vi "XY Sub_VI.vi"(3 "error in (no error)":errorcluster, 5 "XY Cluster In":T1 {"Y Data"."Input"."Tol" min=0.0; "X Data"."Input"."Tol" min=0.0}) -> (0 "error out":errorcluster, 2 "XY Cluster Out":T1 {"Y Data"."Input"."Tol" min=0.0; "X Data"."Input"."Tol" min=0.0})   [LabVIEW 2017]
uses:
  Encoder Cluster.ctl
  <vilib>/myRIO/Common/Instrument Driver Framework/myRIO v1.0/Encoder/typedefs/Encoder Count Direction Enum.ctl
  XY Cluster.ctl
  Motor Status Enum.ctl
  Motion Type Def.ctl
  <vilib>/addons/control/pid/pid.llb/PID Control Input Filter (DBL).vi
  <vilib>/addons/control/pid/pid.llb/PID (DBL).vi
  <vilib>/addons/control/pid/NI_PID_pid.lvlib
  <vilib>/ptbypt/NI_PtbyPt.lvlib
panel:
  out "Data Array":string[][](array[string])
  out "Stop":bool
  out "Y dist > +20":bool
  out "X dist > +20":bool
  out "X V Array":dbl[](array[numeric])
  out "Y V Array":dbl[](array[numeric])
  out "Encoder Output":T4
  out "X&Y Complete":bool
  out "Y PID Output":dbl format="%.2f"
  out "X PID Output":dbl format="%.2f"
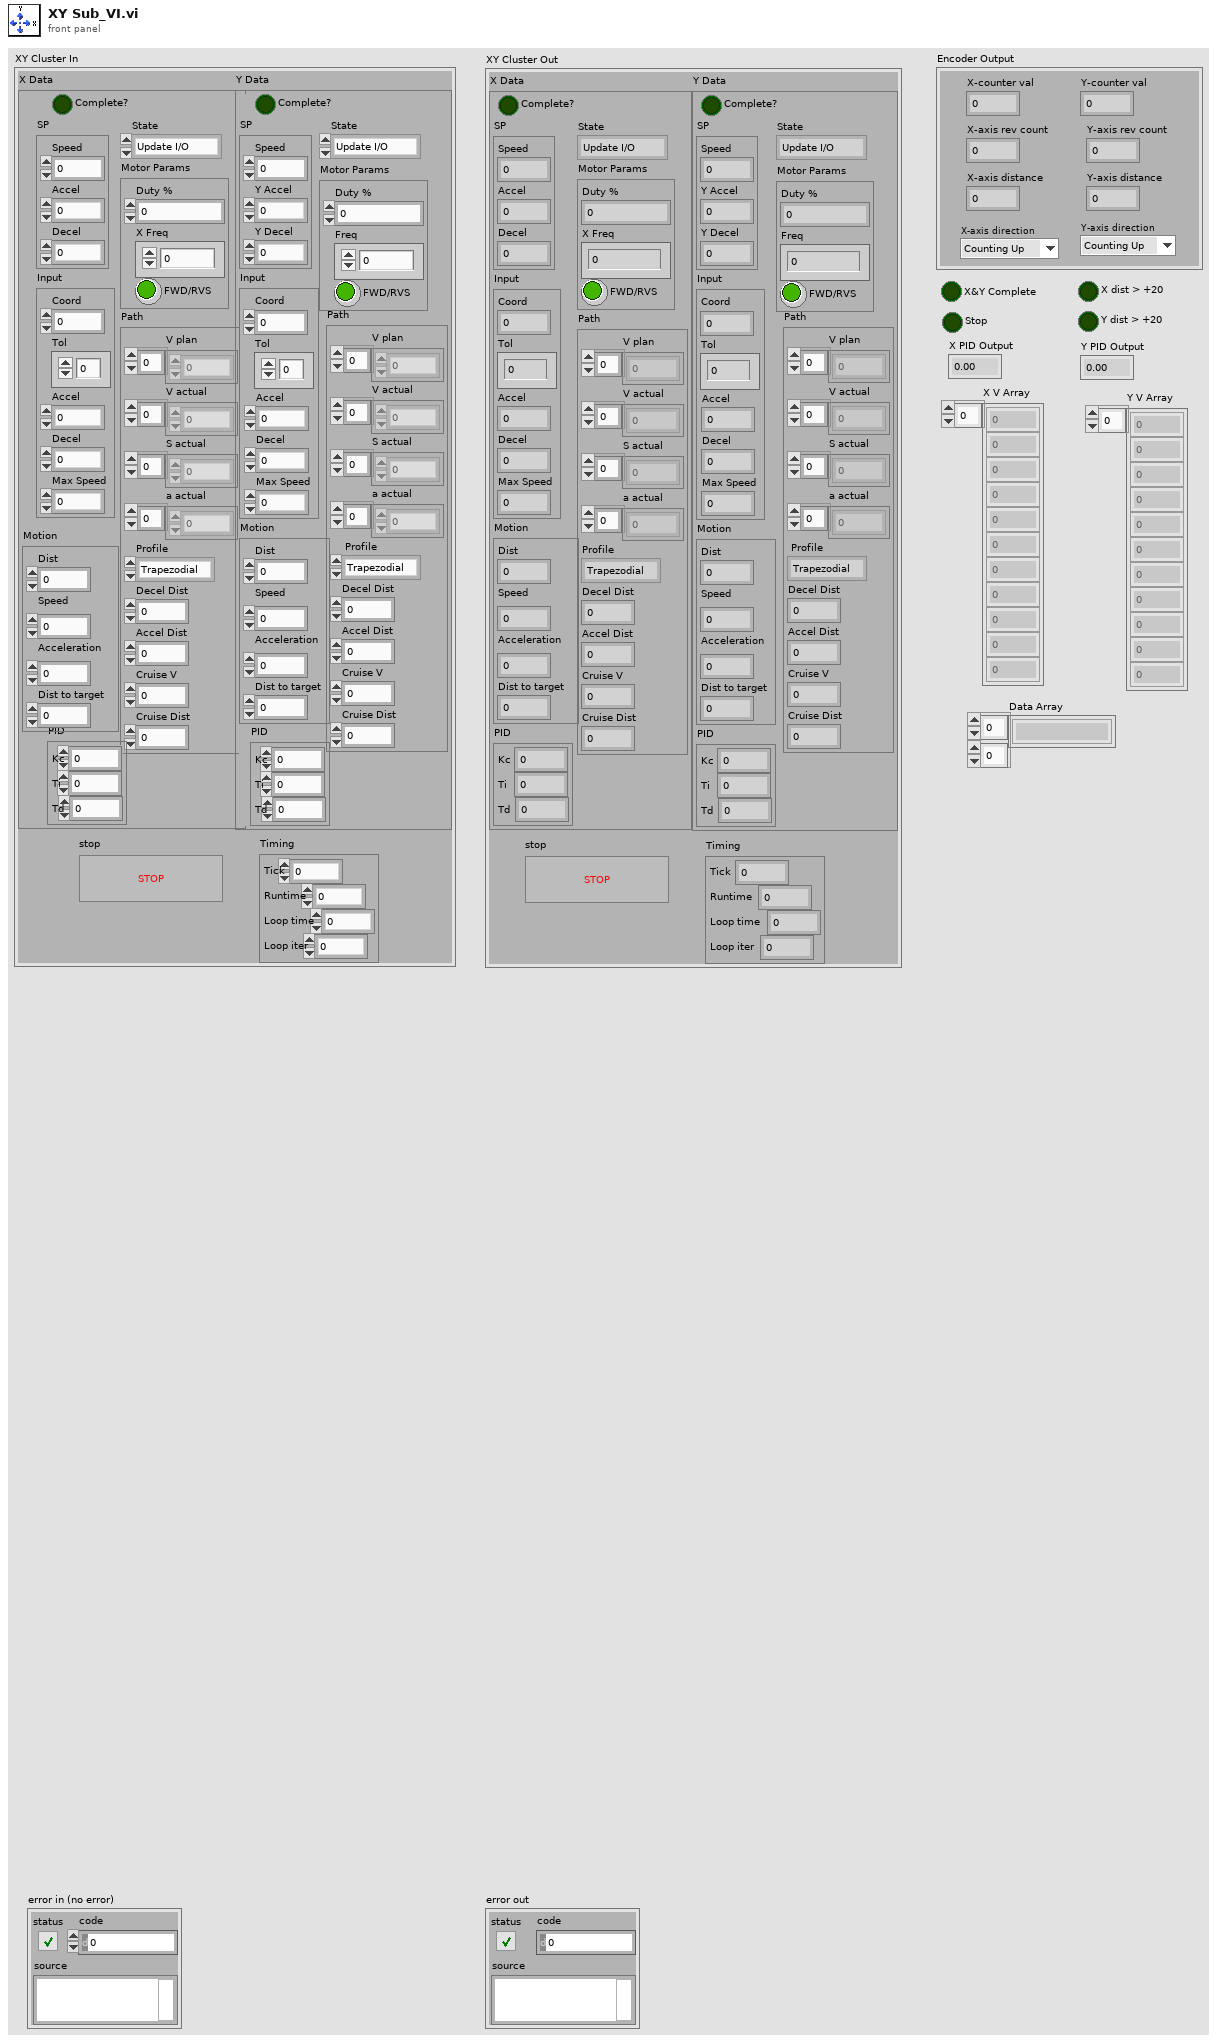
[diagram p1: front panel]
types:
  T1 = typedef "XY Cluster.ctl" = cluster{"X Data":cluster{"Complete?":bool, "Motor Params":cluster{"Duty %":dbl, "X Freq":dbl, "FWD/RVS":bool}, "SP":cluster{"Accel":dbl, "Decel":dbl, "Speed":dbl}, "State":T2, "Input":cluster{"Coord":dbl, "Tol":dbl, "Accel":dbl, "Decel":dbl, "Max Speed":dbl}, "Path":cluster{"V plan":dbl[], "V actual":dbl[], "S actual":dbl[], "a actual":dbl[], "Profile":T3, "Decel Dist":dbl, "Accel Dist":dbl, "Cruise V":dbl, "Cruise Dist":dbl}, "PID":cluster{"Kc":dbl, "Ti":dbl, "Td":dbl}, "Motion":cluster{"Speed":dbl, "Dist":dbl, "Acceleration":dbl, "Dist to target":dbl}}, "Y Data":cluster{"Complete?":bool, "Motor Params":cluster{"Duty %":dbl, "Freq":dbl, "FWD/RVS":bool}, "SP":cluster{"Y Accel":dbl, "Y Decel":dbl, "Speed":dbl}, "State":T2, "Input":cluster{"Coord":dbl, "Tol":dbl, "Accel":dbl, "Decel":dbl, "Max Speed":dbl}, "Path":cluster{"V plan":dbl[], "V actual":dbl[], "S actual":dbl[], "a actual":dbl[], " Profile":T3, "Decel Dist":dbl, "Accel Dist":dbl, "Cruise V":dbl, "Cruise Dist":dbl}, "PID":cluster{"Kc":dbl, "Ti":dbl, "Td":dbl}, "Motion":cluster{"Speed":dbl, "Dist":dbl, "Acceleration":dbl, "Dist to target":dbl}}, "Timing":cluster{"Runtime":dbl, "Loop time":dbl, "Loop iter":i32, "Tick":dbl}, "stop":bool}
  T2 = typedef "Motor Status Enum.ctl" = enum16{"Update I/O", "Stop", "Steady Speed", "Accelerate", "Decelerate", "Drive Motor"}
  T3 = typedef "Motion Type Def.ctl" = enum16{"Trapezodial", "Triangular"}
  T4 = typedef "Encoder Cluster.ctl" = cluster{"Y-axis rev count":dbl, "Y-axis distance":dbl, "X-axis rev count":dbl, "X-axis distance":dbl, "Y-axis direction":T5, "X-axis direction":T5, "X-counter val":i32, "Y-counter val":i32}
  T5 = typedef "Encoder Count Direction Enum.ctl" = enum16{"Counting Up", "Counting Down"}
  T6 = cluster{"Dist to target (mm)":dbl, "Max Speed (mm/s)":dbl, "Max Accel (mm/s^2)":dbl, "Max Decel (mm/s^2)":dbl, "Step Time (s)":dbl}
  T7 = cluster{" Distance target (mm)":dbl, "Max Accel (mm/s^2)":dbl, "Max Decel (mm/s^2)":dbl, "Velocity Limit (mm/s) ":dbl}
  T8 = cluster{"Complete?":bool, "Motor Params":cluster{"Duty %":dbl, "X Freq":dbl, "FWD/RVS":bool}, "SP":cluster{"Accel":dbl, "Decel":dbl, "Speed":dbl}, "State":T2, "Input":cluster{"Coord":dbl, "Tol":dbl, "Accel":dbl, "Decel":dbl, "Max Speed":dbl}, "Path":cluster{"V plan":dbl[], "V actual":dbl[], "S actual":dbl[], "a actual":dbl[], "Profile":T3, "Decel Dist":dbl, "Accel Dist":dbl, "Cruise V":dbl, "Cruise Dist":dbl}, "PID":cluster{"Kc":dbl, "Ti":dbl, "Td":dbl}, "Motion":cluster{"Speed":dbl, "Dist":dbl, "Acceleration":dbl, "Dist to target":dbl}}
  T9 = cluster{"Crusing Time (s)":dbl, "Decel Time (s)":dbl, "Accel Time (s)":dbl, "Total Time (s)":dbl, "Accel Distance (mm)":dbl, "Decel Distance (mm)":dbl, "Crusing Distance (mm)":dbl, "Total Dist (mm)":dbl, "Max Speed (mm/s)":dbl}
  T10 = cluster{"Complete?":bool, "Motor Params":cluster{"Duty %":dbl, "Freq":dbl, "FWD/RVS":bool}, "SP":cluster{"Y Accel":dbl, "Y Decel":dbl, "Speed":dbl}, "State":T2, "Input":cluster{"Coord":dbl, "Tol":dbl, "Accel":dbl, "Decel":dbl, "Max Speed":dbl}, "Path":cluster{"V plan":dbl[], "V actual":dbl[], "S actual":dbl[], "a actual":dbl[], " Profile":T3, "Decel Dist":dbl, "Accel Dist":dbl, "Cruise V":dbl, "Cruise Dist":dbl}, "PID":cluster{"Kc":dbl, "Ti":dbl, "Td":dbl}, "Motion":cluster{"Speed":dbl, "Dist":dbl, "Acceleration":dbl, "Dist to target":dbl}}
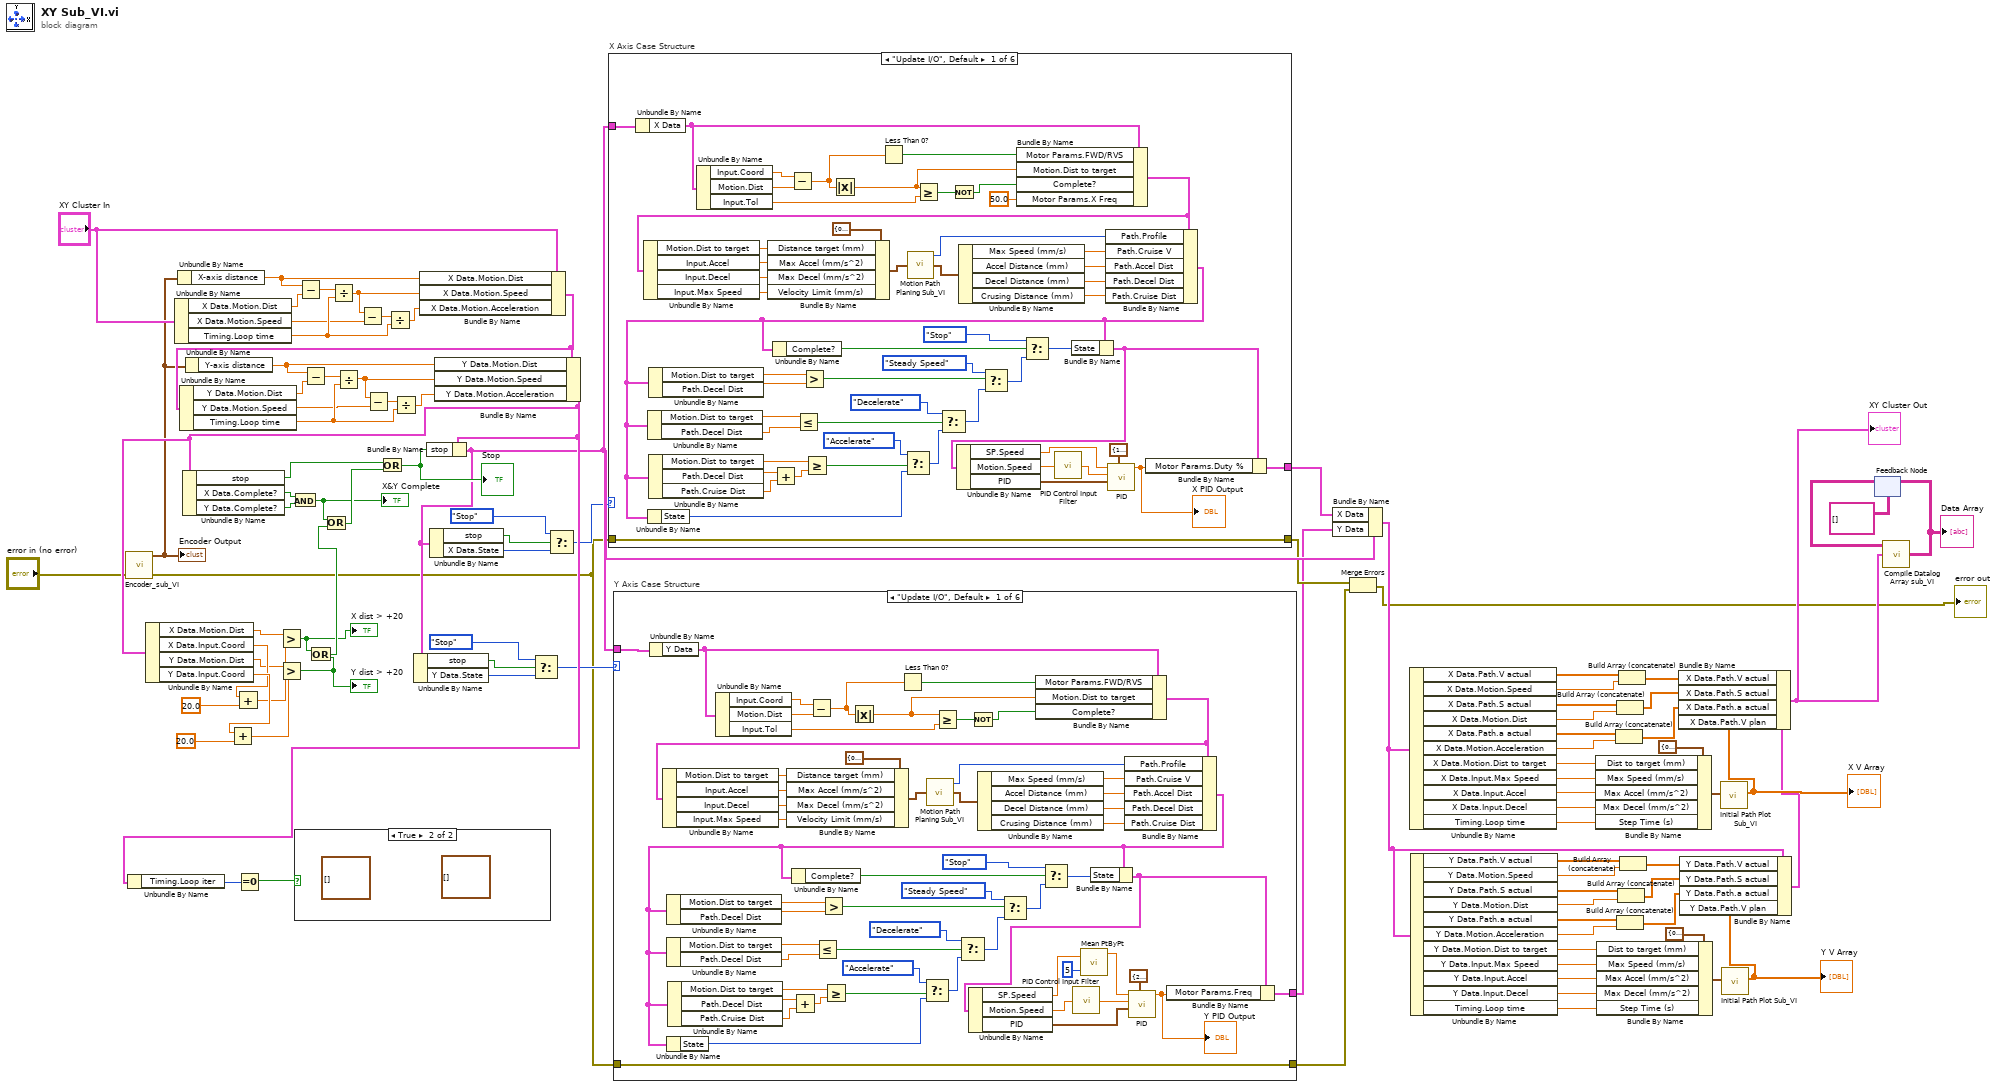
[diagram p0: block diagram]
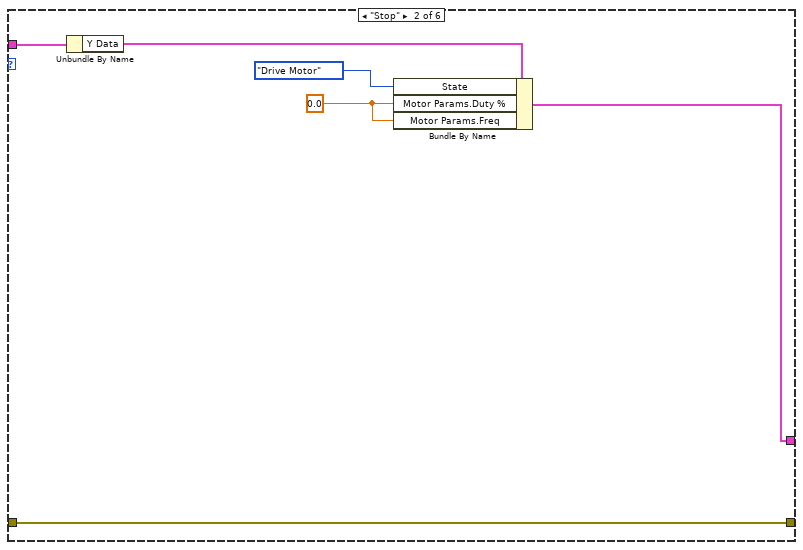
[diagram p3: hidden frame]
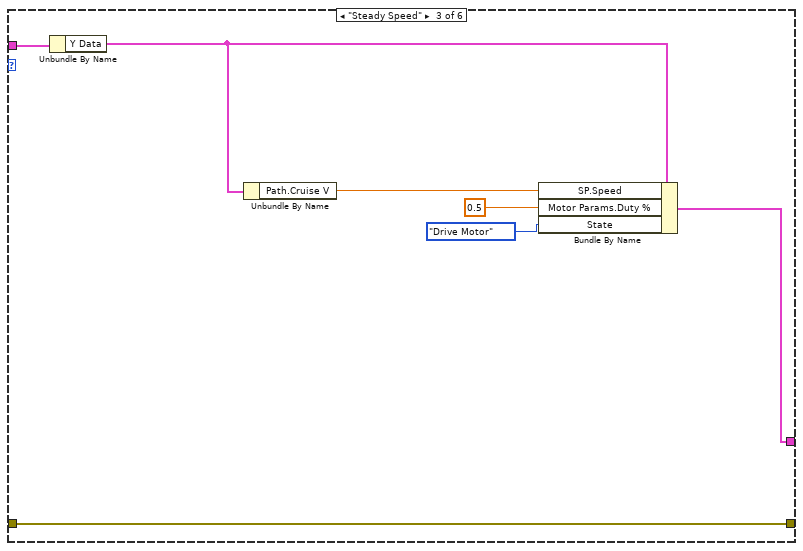
[diagram p4: hidden frame]
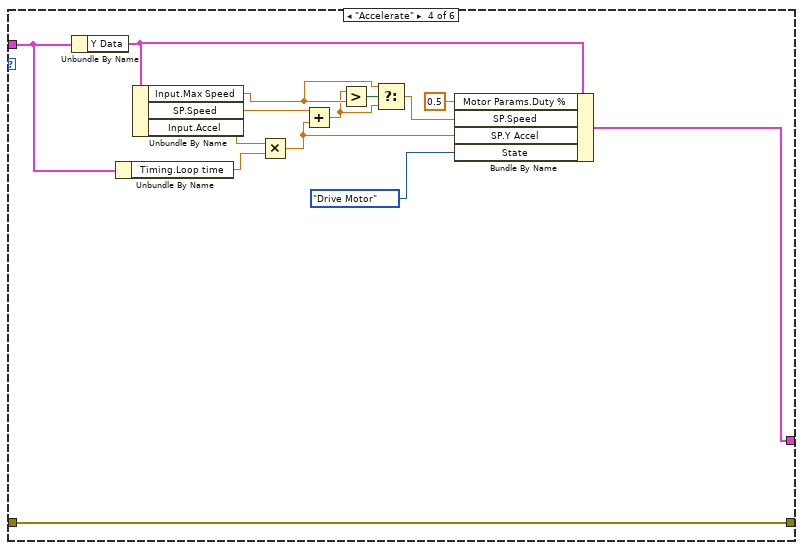
[diagram p5: hidden frame]
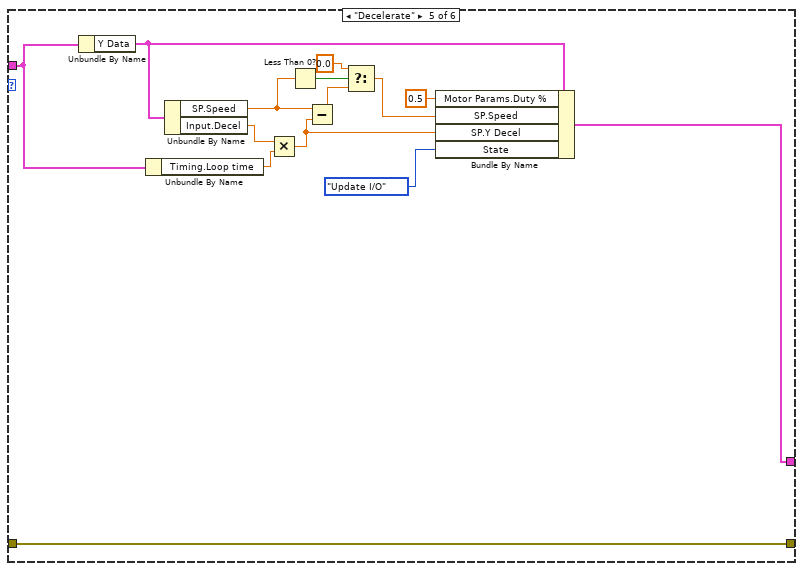
[diagram p6: hidden frame]
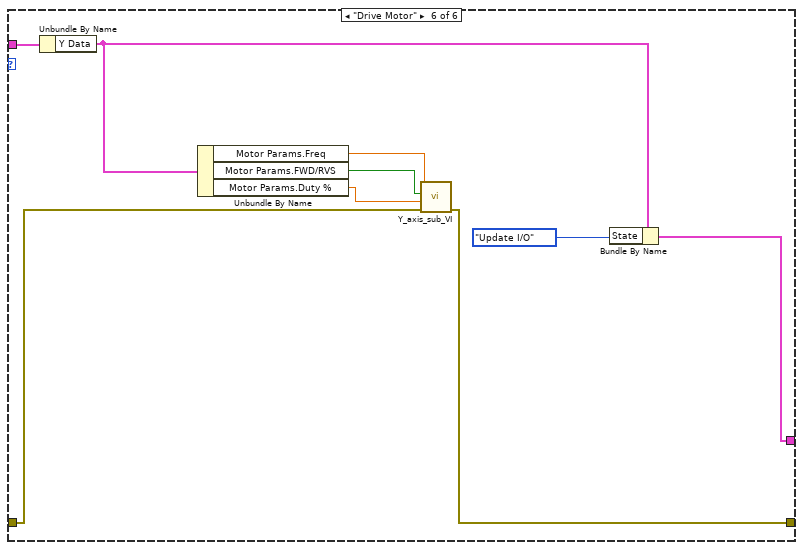
[diagram p7: hidden frame]
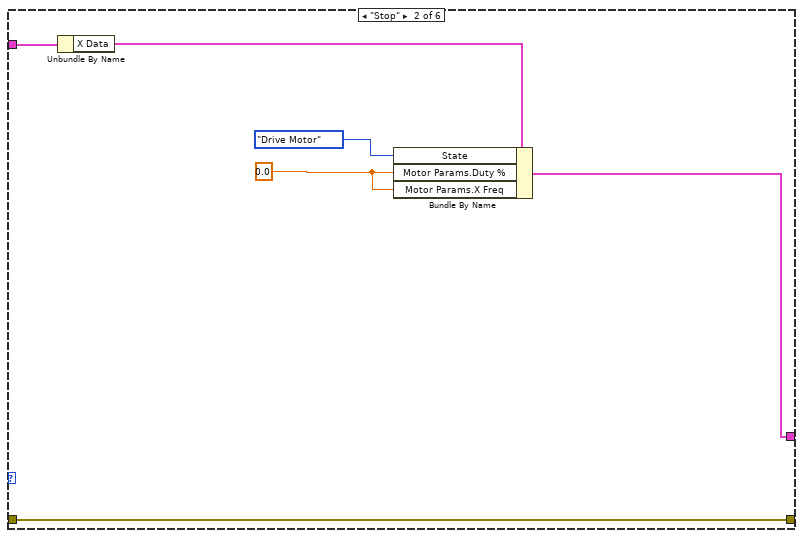
[diagram p8: hidden frame]
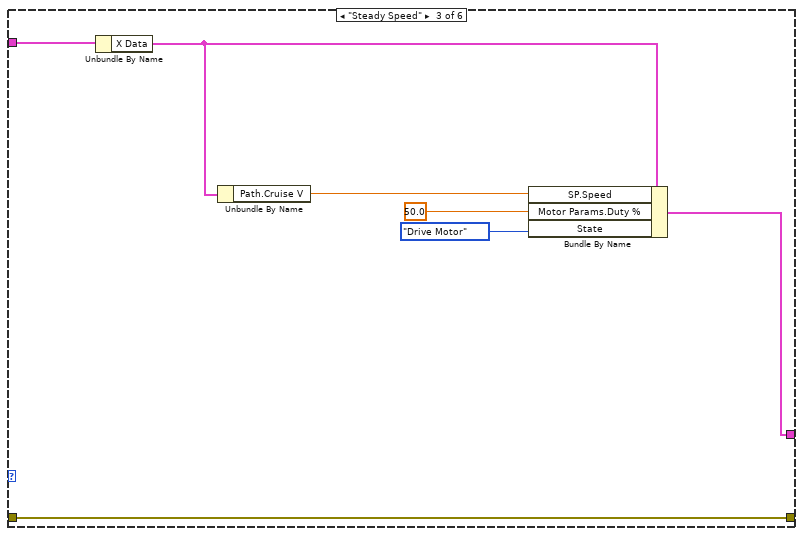
[diagram p9: hidden frame]
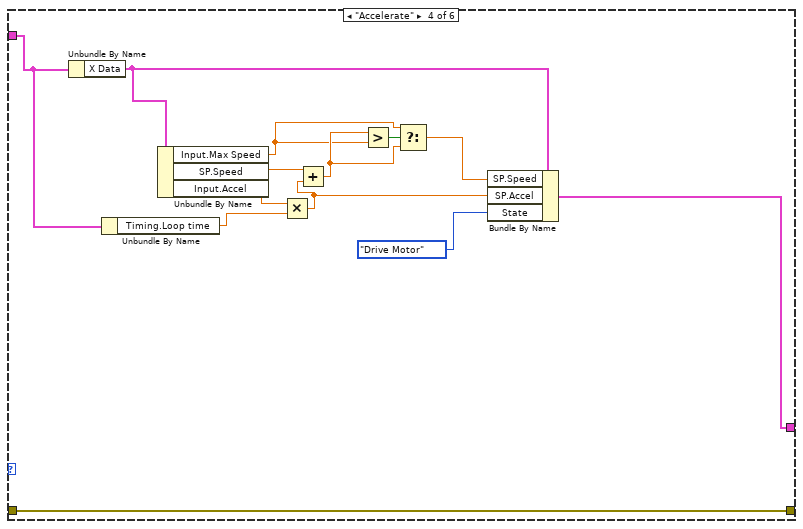
[diagram p10: hidden frame]
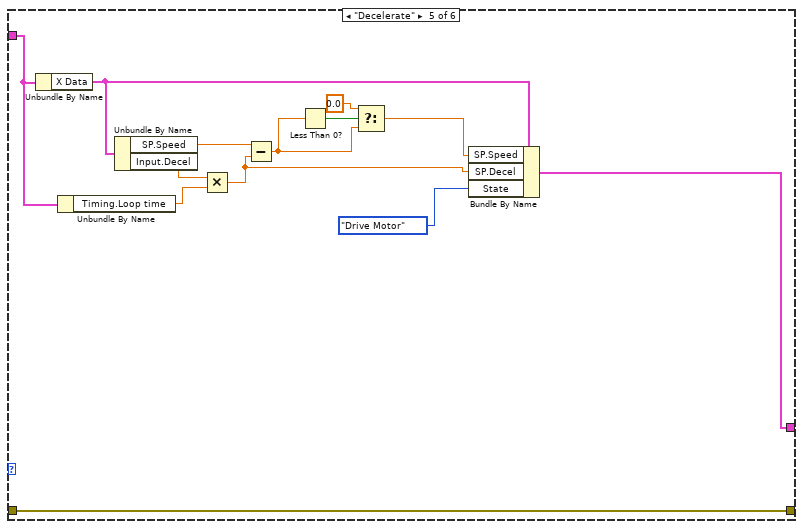
[diagram p11: hidden frame]
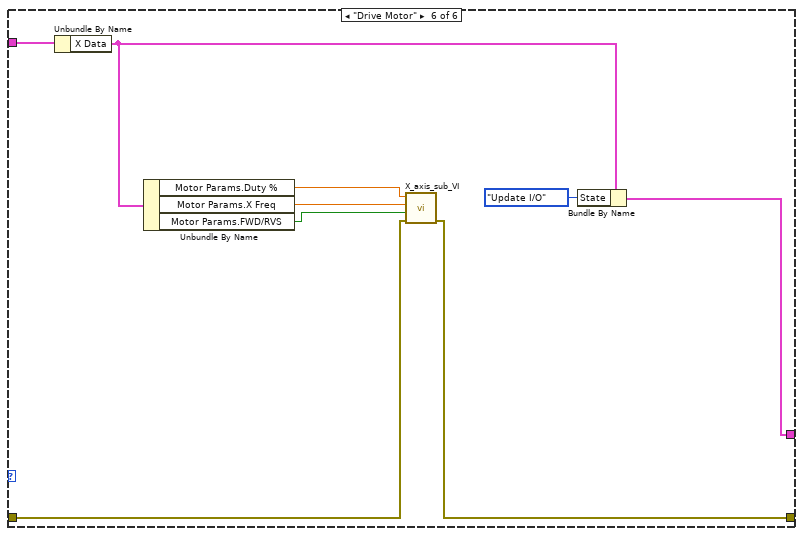
[diagram p12: hidden frame]
diagram:
  n1 = call "Encoder_sub_VI.vi"("error in (no error)"="error in (no error)") -> ("error out"=w22:errorcluster, "Encoder Output"=w12:T4)  [unwired: 9 in]
  "Encoder Output" <- w12
  n2 = Unbundle By Name("XY Cluster In") -> ("X Data.Motion.Dist"=w5:dbl, "X Data.Motion.Speed"=w8:dbl, "Timing.Loop time"=w10:dbl)
  n3 = Unbundle By Name(w12) -> ("X-axis distance"=w4:dbl)
  n4 = Unbundle By Name(w12) -> ("Y-axis distance"=w21:dbl)
  n5 = Subtract(x=w4, y=w5) -> (x-y=w6:dbl)
  n6 = Divide(x=w6, y=w10) -> (x/y=w9:dbl)
  n7 = Subtract(x=w9, y=w8) -> (x-y=w7:dbl)
  n8 = Divide(x=w7, y=w10) -> (x/y=w11:dbl)
  n9 = Bundle By Name(cluster="XY Cluster In", "X Data.Motion.Dist"=w4, "X Data.Motion.Speed"=w9, "X Data.Motion.Acceleration"=w11) -> (w20:T1)
  n10 = Unbundle By Name(w20) -> ("Y Data.Motion.Dist"=w13:dbl, "Y Data.Motion.Speed"=w16:dbl, "Timing.Loop time"=w18:dbl)
  n11 = Subtract(x=w21, y=w13) -> (x-y=w14:dbl)
  n12 = Divide(x=w14, y=w18) -> (x/y=w17:dbl)
  n13 = Subtract(x=w17, y=w16) -> (x-y=w15:dbl)
  n14 = Divide(x=w15, y=w18) -> (x/y=w19:dbl)
  n15 = Bundle By Name(cluster=w20, "Y Data.Motion.Dist"=w21, "Y Data.Motion.Speed"=w17, "Y Data.Motion.Acceleration"=w19) -> (w91:T1)
  n16 = Unbundle By Name(w91) -> ("Timing.Loop iter"=w93:i32)
  n17 = Unbundle By Name(w91) -> ("X Data.Motion.Dist"=w79:dbl, "X Data.Input.Coord"=w86:dbl, "Y Data.Motion.Dist"=w81:dbl, "Y Data.Input.Coord"=w89:dbl)
  n18 = Unbundle By Name(w91) -> ("stop"=w1:bool, "X Data.Complete?"=w38:bool, "Y Data.Complete?"=w39:bool)
  n19 = Add(x=w89, y=20.0) -> (x+y=w90:dbl)
  n20 = Add(x=w86, y=20.0) -> (x+y=w87:dbl)
  n21 = Equal To 0?(x=w93) -> (x = 0?=w92:bool)
  n22 = Greater?(x=w79, y=w87) -> (0:w80:bool)
  "X dist > +20" <- w80
  n23 = Greater?(x=w81, y=w90) -> (0:w84:bool)
  "Y dist > +20" <- w84
  n24 = And(x=w38, y=w39) -> (x .and. y?=w83:bool)
  "X&Y Complete" <- w83
  n25 = case shown="True" w92 {
    frame False {
    }
    frame True {
      (unwired) cluster{"Speed":dbl, "Speed":dbl}[] [] ("History Data")
      (unwired) cluster{"Speed":dbl, "Speed":dbl}[] [] ("History Data")
    }
  }
  n26 = Or(x=w80, y=w84) -> (x .or. y?=w82:bool)
  n27 = Or(x=w83, y=w82) -> (x .or. y?=w94:bool)
  n28 = Or(x=w1, y=w94) -> (x .or. y?=w95:bool)
  "Stop" <- w95
  n29 = Bundle By Name(cluster=w91, "stop"=w95) -> (w77:T1)
  n30 = Unbundle By Name(w77) -> ("stop"=w35:bool, "Y Data.State"=w34:T2)
  n31 = Unbundle By Name(w77) -> ("stop"=w31:bool, "X Data.State"=w30:T2)
  n32 = Select(t=Motor_Status_Enum."Stop", s=w35, f=w34) -> (s? t:f=w37:T2)
  n33 = Select(t=Motor_Status_Enum."Stop", s=w31, f=w30) -> (s? t:f=w33:T2)
  n34 = case "X Axis Case Structure" shown="\"Update I/O\", Default" w33 {
    tunnel: [w119 w156 w161 w175 w183 w191] -> w3
    tunnel: w22 -> [w140 w151 w159 w173 w182 w194]
    tunnel: [w140 w151 w159 w173 w182 w193] -> w25
    tunnel: w77 -> [w120 w153 w162 w174 w185 w198]
    frame "Update I/O", Default {
      n35 = Unbundle By Name(w120) -> ("X Data"=w102:T8)
      n36 = Unbundle By Name(w102) -> ("Input.Coord"=w150:dbl, "Motion.Dist"=w145:dbl, "Input.Tol"=w149:dbl)
      n37 = Subtract(x=w150, y=w145) -> (x-y=w146:dbl)
      n38 = Absolute Value(x=w146) -> (abs(x)=w117:dbl)
      n39 = Less Than 0?(x=w146) -> (x < 0?=w118:bool)
      n40 = Greater Or Equal?(x=w117, y=w149) -> (x >= y?=w148:bool)
      n41 = Not(x=w148) -> (.not. x?=w147:bool)
      n42 = Bundle By Name(cluster=w102, "Motor Params.FWD/RVS"=w118, "Motion.Dist to target"=w117, "Complete?"=w147, "Motor Params.X Freq"=50.0) -> (w115:T8)
      n43 = Unbundle By Name(w115) -> ("Motion.Dist to target"=w116:dbl, "Input.Accel"=w137:dbl, "Input.Decel"=w136:dbl, "Input.Max Speed"=w138:dbl)
      n44 = Bundle By Name(cluster=T7 {" Distance target (mm)"=0.0, "Max Accel (mm/s^2)"=0.0, "Max Decel (mm/s^2)"=0.0, "Velocity Limit (mm/s) "=0.0} ("Motion Planning Inputs"), "Distance target (mm)"=w116, "Max Accel (mm/s^2)"=w137, "Max Decel (mm/s^2)"=w136, "Velocity Limit (mm/s)"=w138) -> (w98:T7)
      n45 = call "Motion Path Planing Sub_VI.vi"("Motion Planning Inputs"=w98) -> ("Motion Profile"=w97:T3, "Motion Planning Outputs"=w96:T9)  [unwired: 5 in]
      n46 = Unbundle By Name(w96) -> ("Max Speed (mm/s)"=w139:dbl, "Accel Distance (mm)"=w134:dbl, "Decel Distance (mm)"=w133:dbl, "Crusing Distance (mm)"=w114:dbl)
      n47 = Bundle By Name(cluster=w115, "Path.Profile"=w97, "Path.Cruise V"=w139, "Path.Accel Dist"=w134, "Path.Decel Dist"=w133, "Path.Cruise Dist"=w114) -> (w109:T8)
      n48 = Unbundle By Name(w109) -> ("Motion.Dist to target"=w111:dbl, "Path.Decel Dist"=w110:dbl)
      n49 = Unbundle By Name(w109) -> ("State"=w131:T2)
      n50 = Unbundle By Name(w109) -> ("Motion.Dist to target"=w113:dbl, "Path.Decel Dist"=w112:dbl)
      n51 = Unbundle By Name(w109) -> ("Motion.Dist to target"=w105:dbl, "Path.Decel Dist"=w108:dbl, "Path.Cruise Dist"=w107:dbl)
      n52 = Unbundle By Name(w109) -> ("Complete?"=w123:bool)
      n53 = Add(x=w108, y=w107) -> (x+y=w106:dbl)
      n54 = Less Or Equal?(x=w111, y=w110) -> (x <= y?=w130:bool)
      n55 = Greater?(x=w113, y=w112) -> (0:w126:bool)
      n56 = Greater Or Equal?(x=w105, y=w106) -> (x >= y?=w104:bool)
      n57 = Select(t=Motor_Status_Enum."Accelerate" ("State"), s=w104, f=w131) -> (s? t:f=w129:T2)
      n58 = Select(t=Motor_Status_Enum."Decelerate" ("State"), s=w130, f=w129) -> (s? t:f=w125:T2)
      n59 = Select(t=Motor_Status_Enum."Steady Speed" ("State"), s=w126, f=w125) -> (s? t:f=w124:T2)
      n60 = Select(t=Motor_Status_Enum."Stop" ("State"), s=w123, f=w124) -> (s? t:f=w121:T2)
      n61 = Bundle By Name(cluster=w109, "State"=w121) -> (w103:T8)
      n62 = Unbundle By Name(w103) -> ("SP.Speed"=w135:dbl, "Motion.Speed"=w143:dbl, "PID"=w142:cluster{"Kc":dbl, "Ti":dbl, "Td":dbl})
      n63 = call-poly <vilib>:"PID Control Input Filter.vi"("input"=w143) -> ("output"=w144:dbl)  [unwired: 4 in]
      n64 = call-poly <vilib>:"PID.vi"("output range"=cluster{"output high":dbl, "output low":dbl} {"output high"=100.0, "output low"=0.0}, "PID gains"=w142, "process variable"=w144, "setpoint"=w135) -> ("output"=w101:dbl)  [unwired: 6 in, 1 out]
      "X PID Output" <- w101
      n65 = Bundle By Name(cluster=w103, "Motor Params.Duty %"=w101) -> (w119:T8)
    }
    frame "Stop" {
      w155 = 0.0
      n66 = Unbundle By Name(w153) -> ("X Data"=w152:T8)
      n67 = Bundle By Name(cluster=w152, "State"=Motor_Status_Enum."Drive Motor", "Motor Params.Duty %"=w155, "Motor Params.X Freq"=w155) -> (w156:T8)
    }
    frame "Steady Speed" {
      n68 = Unbundle By Name(w162) -> ("X Data"=w158:T8)
      n69 = Unbundle By Name(w158) -> ("Path.Cruise V"=w157:dbl)
      n70 = Bundle By Name(cluster=w158, "SP.Speed"=w157, "Motor Params.Duty %"=50.0, "State"=Motor_Status_Enum."Drive Motor") -> (w161:T8)
    }
    frame "Accelerate" {
      n71 = Unbundle By Name(w174) -> ("X Data"=w176:T8)
      n72 = Unbundle By Name(w174) -> ("Timing.Loop time"=w172:dbl)
      n73 = Unbundle By Name(w176) -> ("Input.Max Speed"=w164:dbl, "SP.Speed"=w170:dbl, "Input.Accel"=w169:dbl)
      n74 = Multiply(x=w169, y=w172) -> (x*y=w168:dbl)
      n75 = Add(x=w170, y=w168) -> (x+y=w165:dbl)
      n76 = Greater?(x=w165, y=w164) -> (0:w167:bool)
      n77 = Select(t=w164, s=w167, f=w165) -> (s? t:f=w166:dbl)
      n78 = Bundle By Name(cluster=w176, "SP.Speed"=w166, "SP.Accel"=w168, "State"=Motor_Status_Enum."Drive Motor") -> (w175:T8)
    }
    frame "Decelerate" {
      n79 = Unbundle By Name(w185) -> ("X Data"=w184:T8)
      n80 = Unbundle By Name(w185) -> ("Timing.Loop time"=w189:dbl)
      n81 = Unbundle By Name(w184) -> ("SP.Speed"=w187:dbl, "Input.Decel"=w186:dbl)
      n82 = Multiply(x=w186, y=w189) -> (x*y=w181:dbl)
      n83 = Subtract(x=w187, y=w181) -> (x-y=w177:dbl)
      n84 = Less Than 0?(x=w177) -> (x < 0?=w180:bool)
      n85 = Select(t=0.0, s=w180, f=w177) -> (s? t:f=w179:dbl)
      n86 = Bundle By Name(cluster=w184, "SP.Speed"=w179, "SP.Decel"=w181, "State"=Motor_Status_Enum."Drive Motor") -> (w183:T8)
    }
    frame "Drive Motor" {
      n87 = Unbundle By Name(w198) -> ("X Data"=w192:T8)
      n88 = Unbundle By Name(w192) -> ("Motor Params.Duty %"=w197:dbl, "Motor Params.X Freq"=w196:dbl, "Motor Params.FWD/RVS"=w195:bool)
      n89 = call "X_axis_sub_VI.vi"("error in (no error)"=w194, "FWD/RVS"=w195, "Frequency"=w196, "Duty Cycle %"=w197) -> ("error out"=w193:errorcluster)  [unwired: 7 in]
      n90 = Bundle By Name(cluster=w192, "State"=Motor_Status_Enum."Update I/O") -> (w191:T8)
    }
  }
  n91 = case "Y Axis Case Structure" shown="\"Update I/O\", Default" w37 {
    tunnel: [w208 w260 w265 w280 w290 w298] -> w23
    tunnel: w22 -> [w254 w255 w264 w278 w289 w304]
    tunnel: [w254 w255 w264 w278 w289 w303] -> w26
    tunnel: w77 -> [w253 w257 w266 w279 w292 w302]
    frame "Update I/O", Default {
      n92 = Unbundle By Name(w253) -> ("Y Data"=w207:T10)
      n93 = Unbundle By Name(w207) -> ("Input.Coord"=w252:dbl, "Motion.Dist"=w248:dbl, "Input.Tol"=w251:dbl)
      n94 = Subtract(x=w252, y=w248) -> (x-y=w211:dbl)
      n95 = Absolute Value(x=w211) -> (abs(x)=w224:dbl)
      n96 = Less Than 0?(x=w211) -> (x < 0?=w210:bool)
      n97 = Greater Or Equal?(x=w224, y=w251) -> (x >= y?=w250:bool)
      n98 = Not(x=w250) -> (.not. x?=w249:bool)
      n99 = Bundle By Name(cluster=w207, "Motor Params.FWD/RVS"=w210, "Motion.Dist to target"=w224, "Complete?"=w249) -> (w222:T10)
      n100 = Unbundle By Name(w222) -> ("Motion.Dist to target"=w223:dbl, "Input.Accel"=w240:dbl, "Input.Decel"=w239:dbl, "Input.Max Speed"=w241:dbl)
      n101 = Bundle By Name(cluster=T7 {" Distance target (mm)"=0.0, "Max Accel (mm/s^2)"=0.0, "Max Decel (mm/s^2)"=0.0, "Velocity Limit (mm/s) "=0.0} ("Motion Planning Inputs"), "Distance target (mm)"=w223, "Max Accel (mm/s^2)"=w240, "Max Decel (mm/s^2)"=w239, "Velocity Limit (mm/s)"=w241) -> (w201:T7)
      n102 = call "Motion Path Planing Sub_VI.vi"("Motion Planning Inputs"=w201) -> ("Motion Profile"=w200:T3, "Motion Planning Outputs"=w199:T9)  [unwired: 5 in]
      n103 = Unbundle By Name(w199) -> ("Max Speed (mm/s)"=w242:dbl, "Accel Distance (mm)"=w238:dbl, "Decel Distance (mm)"=w237:dbl, "Crusing Distance (mm)"=w221:dbl)
      n104 = Bundle By Name(cluster=w222, "Path.Profile"=w200, "Path.Cruise V"=w242, "Path.Accel Dist"=w238, "Path.Decel Dist"=w237, "Path.Cruise Dist"=w221) -> (w209:T10)
      n105 = Unbundle By Name(w209) -> ("Motion.Dist to target"=w220:dbl, "Path.Decel Dist"=w219:dbl)
      n106 = Unbundle By Name(w209) -> ("Motion.Dist to target"=w218:dbl, "Path.Decel Dist"=w217:dbl)
      n107 = Unbundle By Name(w209) -> ("State"=w235:T2)
      n108 = Unbundle By Name(w209) -> ("Motion.Dist to target"=w213:dbl, "Path.Decel Dist"=w216:dbl, "Path.Cruise Dist"=w215:dbl)
      n109 = Unbundle By Name(w209) -> ("Complete?"=w227:bool)
      n110 = Add(x=w216, y=w215) -> (x+y=w214:dbl)
      n111 = Less Or Equal?(x=w218, y=w217) -> (x <= y?=w234:bool)
      n112 = Greater?(x=w220, y=w219) -> (0:w230:bool)
      n113 = Greater Or Equal?(x=w213, y=w214) -> (x >= y?=w212:bool)
      n114 = Select(t=Motor_Status_Enum."Accelerate" ("State"), s=w212, f=w235) -> (s? t:f=w233:T2)
      n115 = Select(t=Motor_Status_Enum."Decelerate" ("State"), s=w234, f=w233) -> (s? t:f=w229:T2)
      n116 = Select(t=Motor_Status_Enum."Steady Speed" ("State"), s=w230, f=w229) -> (s? t:f=w228:T2)
      n117 = Select(t=Motor_Status_Enum."Stop" ("State"), s=w227, f=w228) -> (s? t:f=w225:T2)
      n118 = Bundle By Name(cluster=w209, "State"=w225) -> (w206:T10)
      n119 = Unbundle By Name(w206) -> ("SP.Speed"=w204:dbl, "Motion.Speed"=w246:dbl, "PID"=w245:cluster{"Kc":dbl, "Ti":dbl, "Td":dbl})
      n120 = call-poly <vilib>:"PID Control Input Filter.vi"("input"=w246) -> ("output"=w247:dbl)  [unwired: 4 in]
      n121 = call <vilib>:"Mean PtByPt.vi"("x"=w204, "sample length"=5) -> ("mean"=w205:dbl)  [unwired: 2 in, 1 out]
      n122 = call-poly <vilib>:"PID.vi"("output range"=cluster{"output high":dbl, "output low":dbl} {"output high"=23000.0, "output low"=0.0}, "PID gains"=w245, "process variable"=w247, "setpoint"=w205) -> ("output"=w243:dbl)  [unwired: 6 in, 1 out]
      "Y PID Output" <- w243
      n123 = Bundle By Name(cluster=w206, "Motor Params.Freq"=w243) -> (w208:T10)
    }
    frame "Stop" {
      w259 = 0.0
      n124 = Unbundle By Name(w257) -> ("Y Data"=w256:T10)
      n125 = Bundle By Name(cluster=w256, "State"=Motor_Status_Enum."Drive Motor", "Motor Params.Duty %"=w259, "Motor Params.Freq"=w259) -> (w260:T10)
    }
    frame "Steady Speed" {
      n126 = Unbundle By Name(w266) -> ("Y Data"=w262:T10)
      n127 = Unbundle By Name(w262) -> ("Path.Cruise V"=w261:dbl)
      n128 = Bundle By Name(cluster=w262, "SP.Speed"=w261, "Motor Params.Duty %"=0.5, "State"=Motor_Status_Enum."Drive Motor") -> (w265:T10)
    }
    frame "Accelerate" {
      n129 = Unbundle By Name(w279) -> ("Y Data"=w281:T10)
      n130 = Unbundle By Name(w279) -> ("Timing.Loop time"=w277:dbl)
      n131 = Unbundle By Name(w281) -> ("Input.Max Speed"=w269:dbl, "SP.Speed"=w275:dbl, "Input.Accel"=w274:dbl)
      n132 = Multiply(x=w274, y=w277) -> (x*y=w273:dbl)
      n133 = Add(x=w275, y=w273) -> (x+y=w268:dbl)
      n134 = Greater?(x=w268, y=w269) -> (0:w271:bool)
      n135 = Select(t=w269, s=w271, f=w268) -> (s? t:f=w270:dbl)
      n136 = Bundle By Name(cluster=w281, "Motor Params.Duty %"=0.5, "SP.Speed"=w270, "SP.Y Accel"=w273, "State"=Motor_Status_Enum."Drive Motor") -> (w280:T10)
    }
    frame "Decelerate" {
      n137 = Unbundle By Name(w292) -> ("Y Data"=w291:T10)
      n138 = Unbundle By Name(w292) -> ("Timing.Loop time"=w295:dbl)
      n139 = Unbundle By Name(w291) -> ("SP.Speed"=w285:dbl, "Input.Decel"=w293:dbl)
      n140 = Multiply(x=w293, y=w295) -> (x*y=w288:dbl)
      n141 = Less Than 0?(x=w285) -> (x < 0?=w286:bool)
      n142 = Subtract(x=w285, y=w288) -> (x-y=w282:dbl)
      n143 = Select(t=0.0, s=w286, f=w282) -> (s? t:f=w284:dbl)
      n144 = Bundle By Name(cluster=w291, "Motor Params.Duty %"=0.5, "SP.Speed"=w284, "SP.Y Decel"=w288, "State"=Motor_Status_Enum."Update I/O") -> (w290:T10)
    }
    frame "Drive Motor" {
      n145 = Unbundle By Name(w302) -> ("Y Data"=w299:T10)
      n146 = Unbundle By Name(w299) -> ("Motor Params.Freq"=w301:dbl, "Motor Params.FWD/RVS"=w300:bool, "Motor Params.Duty %"=w296:dbl)
      n147 = call "Y_axis_sub_VI.vi"("error in (no error)"=w304, "Duty Cycle"=w296, "FWD/RVS"=w300, "Frequency"=w301) -> ("error out"=w303:errorcluster)  [unwired: 7 in]
      n148 = Bundle By Name(cluster=w299, "State"=Motor_Status_Enum."Update I/O") -> (w298:T10)
    }
  }
  n149 = Bundle By Name(cluster=w77, "X Data"=w3, "Y Data"=w23) -> (w72:T1)
  n150 = Merge Errors(w25, w26) -> (→"error out":errorcluster)
  n151 = Unbundle By Name(w72) -> ("X Data.Path.V actual"=w40:dbl[], "X Data.Motion.Speed"=w41:dbl, "X Data.Path.S actual"=w44:dbl[], "X Data.Motion.Dist"=w45:dbl, "X Data.Path.a actual"=w46:dbl[], "X Data.Motion.Acceleration"=w47:dbl, "X Data.Motion.Dist to target"=w51:dbl, "X Data.Input.Max Speed"=w52:dbl, "X Data.Input.Accel"=w53:dbl, "X Data.Input.Decel"=w54:dbl, "Timing.Loop time"=w55:dbl)
  n152 = Unbundle By Name(w72) -> ("Y Data.Path.V actual"=w56:dbl[], "Y Data.Motion.Speed"=w57:dbl, "Y Data.Path.S actual"=w60:dbl[], "Y Data.Motion.Dist"=w61:dbl, "Y Data.Path.a actual"=w62:dbl[], "Y Data.Motion.Acceleration"=w63:dbl, "Y Data.Motion.Dist to target"=w67:dbl, "Y Data.Input.Max Speed"=w68:dbl, "Y Data.Input.Accel"=w69:dbl, "Y Data.Input.Decel"=w70:dbl, "Timing.Loop time"=w71:dbl)
  n153 = Bundle By Name(cluster=T6 {"Dist to target (mm)"=0.0, "Max Speed (mm/s)"=0.0, "Max Accel (mm/s^2)"=0.0, "Max Decel (mm/s^2)"=0.0, "Step Time (s)"=0.0} ("Motion Inputs"), "Dist to target (mm)"=w51, "Max Speed (mm/s)"=w52, "Max Accel (mm/s^2)"=w53, "Max Decel (mm/s^2)"=w54, "Step Time (s)"=w55) -> (w49:T6)
  n154 = Bundle By Name(cluster=T6 {"Dist to target (mm)"=0.0, "Max Speed (mm/s)"=0.0, "Max Accel (mm/s^2)"=0.0, "Max Decel (mm/s^2)"=0.0, "Step Time (s)"=0.0} ("Motion Inputs"), "Dist to target (mm)"=w67, "Max Speed (mm/s)"=w68, "Max Accel (mm/s^2)"=w69, "Max Decel (mm/s^2)"=w70, "Step Time (s)"=w71) -> (w65:T6)
  n155 = Build Array (concatenate)(w46, w47) -> (w48:dbl[])
  n156 = Build Array (concatenate)(w44, w45) -> (w43:dbl[])
  n157 = Build Array (concatenate)(w62, w63) -> (w64:dbl[])
  n158 = Build Array (concatenate)(w60, w61) -> (w59:dbl[])
  n159 = Build Array (concatenate)(w40, w41) -> (w42:dbl[])
  n160 = Build Array (concatenate)(w56, w57) -> (w58:dbl[])
  n161 = call "Initial Path Plot Sub_VI.vi"("Motion Inputs"=w49) -> ("Velocity Array"=w75:dbl[])  [unwired: 7 in, 3 out]
  "X V Array" <- w75
  n162 = call "Initial Path Plot Sub_VI.vi"("Motion Inputs"=w65) -> ("Velocity Array"=w74:dbl[])  [unwired: 7 in, 3 out]
  "Y V Array" <- w74
  n163 = Bundle By Name(cluster=w72, "Y Data.Path.V actual"=w58, "Y Data.Path.S actual"=w59, "Y Data.Path.a actual"=w64, "Y Data.Path.V plan"=w74) -> (w73:T1)
  n164 = Bundle By Name(cluster=w73, "X Data.Path.V actual"=w42, "X Data.Path.S actual"=w43, "X Data.Path.a actual"=w48, "X Data.Path.V plan"=w75) -> (w78:T1)
  "XY Cluster Out" <- w78
  n165 = feedback #1(string[][] [] ("Initialised Array")) -> (w28:string[][])
  n166 = call "Compile Datalog Array sub_VI.vi"("XY Cluster"=w78, "Initialised Array"=w28) -> ("Data Array"=w27:string[][])  [unwired: 1 in]
  "Data Array" <- w27
  n167 = feedback-in #1(w27) -> ()
